vi "s_InitializeMotor.vi"(2 "Error In":errorcluster, 3 "Servo Controller  ID":i32, 4 "Motor Reference In":refnum<k7>) -> (0 "Error Out":errorcluster, 1 "Motor Reference":refnum<k7>)   [LabVIEW 2014]
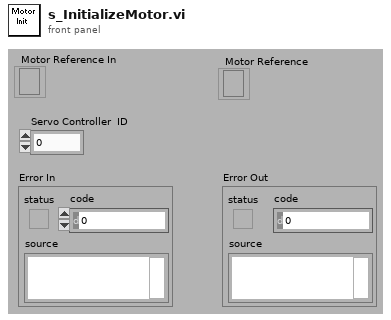
[diagram p1: front panel]
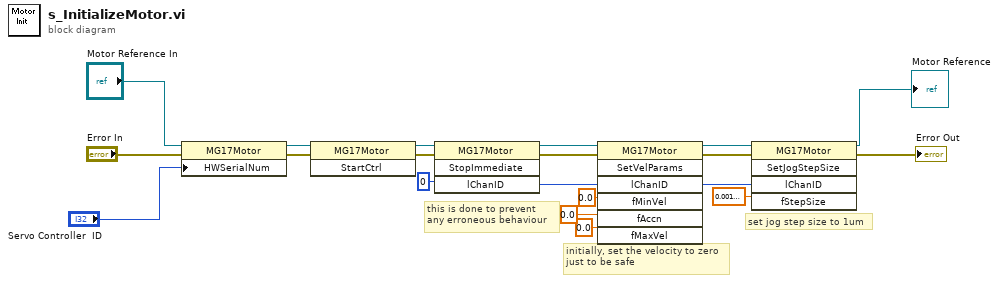
[diagram p0: block diagram]
diagram:
  # "set jog step size to 1um"
  # "initially, set the velocity to zero\njust to be safe"
  # "this is done to prevent \nany erroneous behaviour"
  n1 = property class="MG17Motor"(reference="Motor Reference In", error in="Error In", "HWSerialNum"="Servo Controller  ID") -> (reference out=w16:refnum<k7>, error out=w15:errorcluster)
  n2 = invoke class="MG17Motor" method="StartCtrl"(reference=w16, error in=w15) -> (reference out=w18:refnum<k7>, error out=w19:errorcluster)  [unwired: 1 in, 1 out]
  n3 = invoke class="MG17Motor" method="StopImmediate"(reference=w18, error in=w19, "lChanID"=0) -> (reference out=w9:refnum<k7>, error out=w8:errorcluster, "lChanID"=w1:i32)  [unwired: 1 in, 1 out]
  n4 = invoke class="MG17Motor" method="SetVelParams"(reference=w9, error in=w8, "lChanID"=w1, "fMinVel"=sgl 0.0, "fAccn"=sgl 0.0, "fMaxVel"=sgl 0.0) -> (reference out=w3:refnum<k7>, error out=w5:errorcluster, "lChanID"=w7:i32)  [unwired: 1 in, 4 out]
  n5 = invoke class="MG17Motor" method="SetJogStepSize"(reference=w3, error in=w5, "lChanID"=w7, "fStepSize"=sgl 0.001) -> (reference out=→"Motor Reference":refnum<k7>, error out=→"Error Out":errorcluster)  [unwired: 1 in, 3 out]
